vi "peg-in-hole Test with points and cloud.vi"() -> ()   [LabVIEW 2013]
uses:
  ROS/Code/SubVIs/BaxterSide.ctl
  <vilib>/Utility/config.llb/Read Key (String).vi
  Arm Globals.vi
  <vilib>/Utility/file.llb/Write To Spreadsheet File (DBL).vi
  <vilib>/Utility/config.llb/NI_LVConfig.lvlib
panel:
  out "time":dbl=251572.85700000002
  out "start":u32
  in  "Cloud File":path=path "C:/Program Files/Labview/user.lib/ROSforLV_0.1/Devices/Baxter/NIST2/Peg-in-hole/cloud.script"
  out "Array":cluster{dbl, dbl, dbl, dbl, dbl, dbl}[](array[cluster]) {"?" format="%.6f"}
  in  "Peg Size":dbl=3.0
  in  "Midpoint Name":string="hm"
  in  "h2 Name":string="h2"
  in  "h1 Name":string="h1"
  out "Times":dbl[](array[numeric]) format="%.1f"
  out "Status":string
  in  "Stop":bool
  out "error out":errorcluster
  # "as in Positions.cfg"
  # "Data is saved automatically at end of run\nSet peg size first"
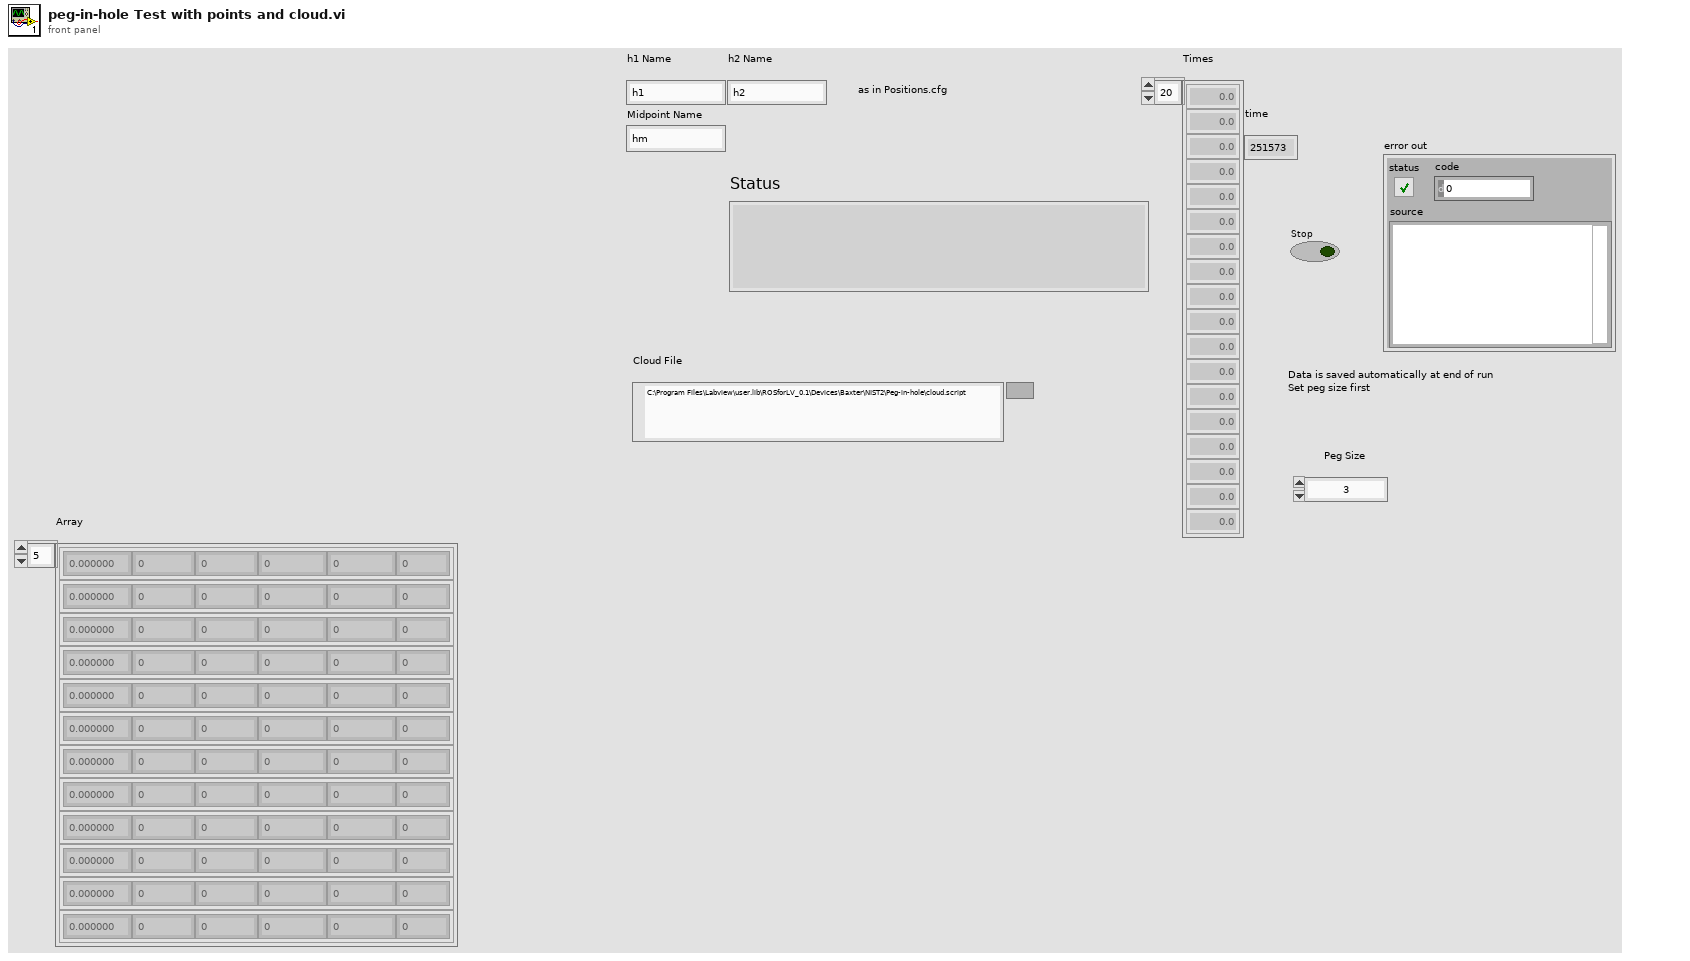
[diagram p1: front panel]
types:
  T1 = typedef "BaxterSide.ctl" = enum16{"left", "right"}
  T2 = typedef "NI_LVConfig.lvlib/Config Data RefNum.ctl" = refnum<k1>
  T3 = typedef "NI_Matrix.lvlib/RealMatrix.ctl" = dbl[][]
  T4 = cluster{"X":dbl, "Y":dbl, "Z":dbl, "Roll":dbl, "Pitch":dbl, "Yaw":dbl}
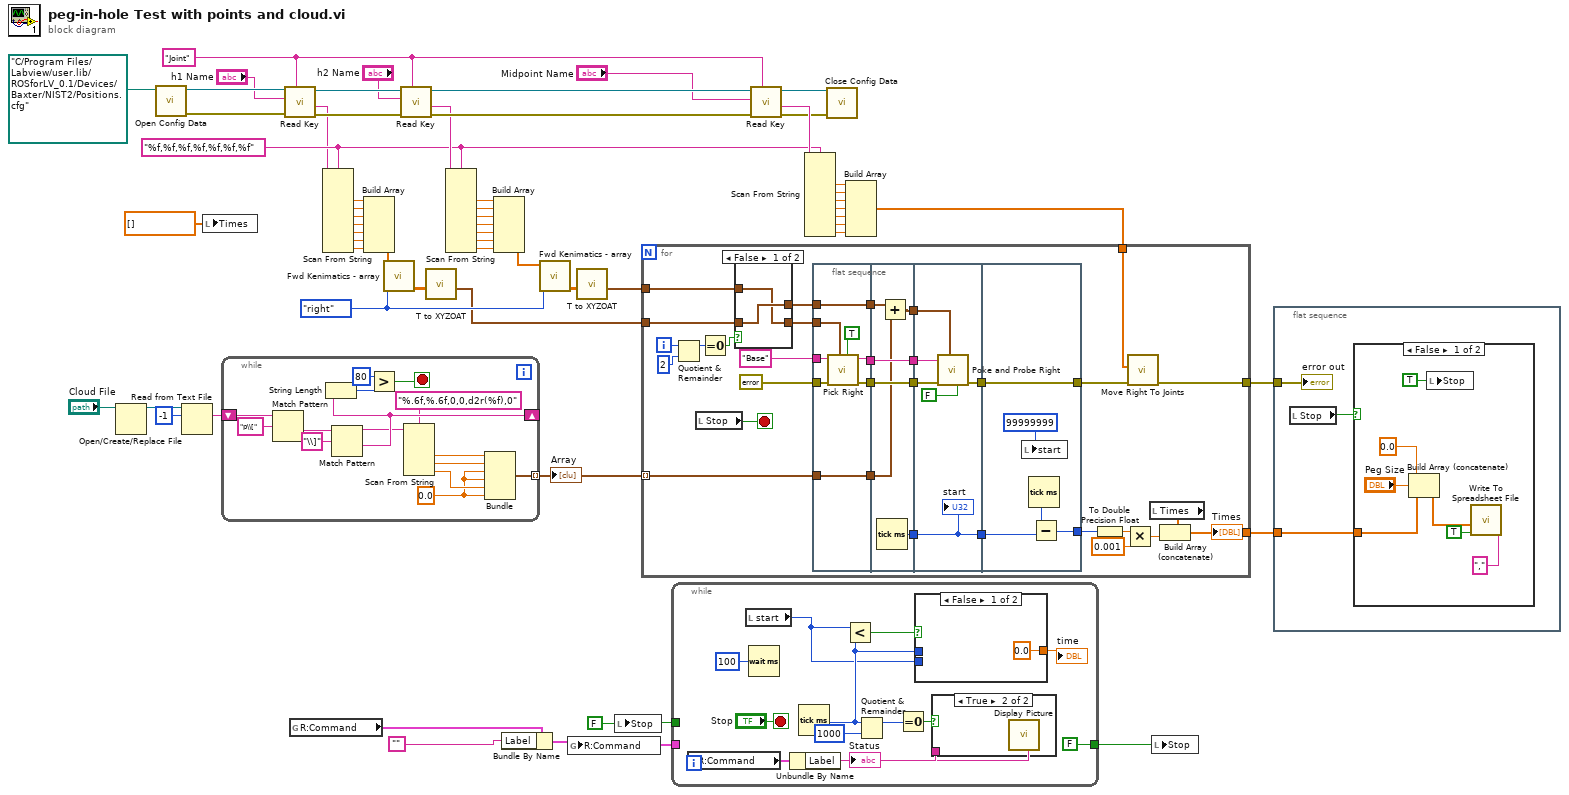
[diagram p0: block diagram]
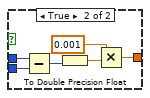
[diagram p3: hidden frame]
diagram:
  w31 = BaxterSide."right" ("Side")
  w15 = "%f,%f,%f,%f,%f,%f,%f" ("format string")
  w22 = "Joint" ("section")
  w58 = FALSE ("Stop")
  n1 = Open/Create/Replace File(file path (use dialog)="Cloud File") -> (refnum out=w5:refnum<file>)  [unwired: 5 in, 2 out]
  n2 = call <vilib>:"Open Config Data.vi"("configuration file path"=path "C:/Program Files/Labview/user.lib/ROSforLV_0.1/Devices/Baxter/NIST2/Positions.cfg") -> ("error out"=w51:errorcluster, "refnum"=w52:T2)  [unwired: 8 in, 1 out]
  n3 = Read from Text File(file (use dialog)=w5, count=-1) -> (text=w3:string)  [unwired: 2 in, 3 out]
  n4 = local write "Times"(dbl[] [] ("Times")) -> ()
  n5 = while {
    shift-right: [w68] -> _
    shift-left: w3 -> [w60]
    tunnel: [w64] -> w1 mode=indexing
    stop <- w72 stop-if-true
    w61 = 0.0
    n6 = Match Pattern(string=w60, regular expression="p\\[") -> (after substring=w70:string)  [unwired: 1 in, 3 out]
    n7 = Match Pattern(string=w70, regular expression="\\]") -> (before substring=w67:string, after substring=w68:string)  [unwired: 1 in, 2 out]
    n8 = String Length(string=w68) -> (length=w74:i32)
    n9 = Greater?(x=80, y=w74) -> (0:w72:bool)
    n10 = Scan From String(format string="%.6f,%.6f,0,0,d2r(%f),0", input string=w67) -> (output 1=w65:dbl, output 2=w63:dbl, output 3=w62:dbl)  [unwired: 5 in, 3 out]
    n11 = Bundle(w65, w63, w61, w61, w62, w61) -> (w64:cluster{dbl, dbl, dbl, dbl, dbl, dbl})  [unwired: 1 in]
  }
  "Array" <- w1
  n12 = call-poly <vilib>:"Read Key.vi"("section"=w22, "error in (no error)"=w51, "key"="h1 Name", "refnum"=w52) -> ("error out"=w25:errorcluster, "value"=w9:string, "refnum out"=w26:T2)  [unwired: 4 in, 1 out]
  n13 = global read "Arm Globals.vi" "R:Command"() -> (w54:cluster{"Label":string, "Angles":dbl[]})
  n14 = Scan From String(format string=w15, input string=w9) -> (output 1=w50:dbl, output 2=w49:dbl, output 3=w48:dbl, output 4=w47:dbl, output 5=w46:dbl, output 6=w45:dbl, output 7=w44:dbl)  [unwired: 9 in, 3 out]
  n15 = Build Array(w50, w49, w48, w47, w46, w45, w44) -> (w32:dbl[])
  n16 = call "Fwd Kenimatics - array.vi"("Side"=w31, "Joints"=w32) -> ("Matrix"=w30:T3)  [unwired: 8 in, 1 out]
  n17 = call-poly <vilib>:"Read Key.vi"("section"=w22, "error in (no error)"=w25, "key"="h2 Name", "refnum"=w26) -> ("error out"=w23:errorcluster, "value"=w16:string, "refnum out"=w24:T2)  [unwired: 4 in, 1 out]
  n18 = call "T to XYZOAT.vi"("T"=w30) -> ("XYZOAT"=w28:T4)  [unwired: 10 in]
  n19 = Scan From String(format string=w15, input string=w16) -> (output 1=w21:dbl, output 2=w20:dbl, output 3=w19:dbl, output 4=w18:dbl, output 5=w17:dbl, output 6=w12:dbl, output 7=w11:dbl)  [unwired: 9 in, 3 out]
  n20 = Build Array(w21, w20, w19, w18, w17, w12, w11) -> (w13:dbl[])
  n21 = Bundle By Name(cluster=w54, "Label"="") -> (w56:cluster{"Label":string, "Angles":dbl[]})
  n22 = call "Fwd Kenimatics - array.vi"("Side"=w31, "Joints"=w13) -> ("Matrix"=w29:T3)  [unwired: 8 in, 1 out]
  n23 = global write "Arm Globals.vi" "R:Command"(w56) -> ()
  n24 = call "T to XYZOAT.vi"("T"=w29) -> ("XYZOAT"=w27:T4)  [unwired: 10 in]
  n25 = local write "Stop"(w58) -> ()
  n26 = while {
    tunnel: w56 -> [_]
    tunnel: [FALSE] -> w57
    tunnel: w58 -> [_]
    stop <- "Stop" stop-if-true
    n27 = global read "Arm Globals.vi" "R:Command"() -> (w86:cluster{"Label":string, "Angles":dbl[]})
    n28 = local read "start"() -> (w77:u32)
    n29 = Wait (ms)(milliseconds to wait=u32 100) -> ()  [unwired: 1 out]
    n30 = Unbundle By Name(w86) -> ("Label"=w80:string)
    "Status" <- w80
    n31 = Tick Count (ms)() -> (millisecond timer value=w78:u32)
    n32 = Less?(x=w77, y=w78) -> (x < y?=w79:bool)
    n33 = Quotient & Remainder(x=w78, y=u32 1000) -> (x-y*floor(x/y)=w82:u32)  [unwired: 1 out]
    n34 = Equal To 0?(x=w82) -> (x = 0?=w81:bool)
    n35 = case shown="False" w79 {
      tunnel: w78 -> [_ w93]
      tunnel: w77 -> [_ w92]
      tunnel: [0.0 w88] -> w76
      frame False {
      }
      frame True {
        n36 = Subtract(x=w93, y=w92) -> (x-y=w91:u32)
        n37 = To Double Precision Float(number=w91) -> (double precision float=w90:dbl)
        n38 = Multiply(x=0.001, y=w90) -> (x*y=w88:dbl)
      }
    }
    "time" <- w76
    n39 = case shown="True" w81 {
      tunnel: w80 -> [_ w94]
      frame False {
      }
      frame True {
        n40 = call "Display Picture.vi"("Comment"=w94) -> ()  [unwired: 10 in, 1 out]
      }
    }
  }
  n41 = call-poly <vilib>:"Read Key.vi"("section"=w22, "error in (no error)"=w23, "key"="Midpoint Name", "refnum"=w24) -> ("error out"=w34:errorcluster, "value"=w36:string, "refnum out"=w35:T2)  [unwired: 4 in, 1 out]
  n42 = Scan From String(format string=w15, input string=w36) -> (output 1=w43:dbl, output 2=w42:dbl, output 3=w41:dbl, output 4=w40:dbl, output 5=w39:dbl, output 6=w38:dbl, output 7=w37:dbl)  [unwired: 9 in, 3 out]
  n43 = call <vilib>:"Close Config Data.vi"("error in (no error)"=w34, "refnum"=w35) -> ()  [unwired: 8 in, 2 out]
  n44 = Build Array(w43, w42, w41, w40, w39, w38, w37) -> (w14:dbl[])
  n45 = for {
    tunnel: [w106] -> w59
    tunnel: w27 -> [w118]
    tunnel: w28 -> [w119]
    tunnel: w14 -> [w100]
    tunnel: [w98] -> w6
    tunnel: w1 -> [w96] mode=indexing
    i -> [w123]
    stop <- w99 stop-if-true
    n46 = Quotient & Remainder(x=w123, y=2) -> (x-y*floor(x/y)=w121:i32)  [unwired: 1 out]
    n47 = local read "Stop"() -> (w99:bool)
    n48 = Equal To 0?(x=w121) -> (x = 0?=w120:bool)
    n49 = case shown="False" w120 {
      tunnel: w119 -> [w127 w129]
      tunnel: [w126 w129] -> w113
      tunnel: w118 -> [w126 w128]
      tunnel: [w127 w128] -> w111
      frame False {
      }
      frame True {
      }
    }
    n50 = flat-sequence {
      tunnel: "Base" ("Location Out") -> [w135]
      tunnel: errorcluster {"status"=FALSE, "code"=0, "source"=""} ("error in") -> [w137]
      tunnel: [w136] -> w117
      tunnel: [w134] -> w115
      tunnel: w113 -> [w133]
      tunnel: [w132] -> w112
      tunnel: w111 -> [w132]
      tunnel: [w131] -> w97
      tunnel: w96 -> [w131]
      tunnel: w117 -> [w143]
      tunnel: [w143] -> w116
      tunnel: w115 -> [w142]
      tunnel: [w142] -> w114
      tunnel: w112 -> [w140]
      tunnel: [w141] -> w108
      tunnel: w97 -> [w139]
      tunnel: [w138] -> w95
      tunnel: [w146] -> w110
      tunnel: w116 -> [w149]
      tunnel: w114 -> [w148]
      tunnel: [w145] -> w109
      tunnel: w108 -> [w145]
      tunnel: w95 -> [w147]
      tunnel: w110 -> [w152]
      tunnel: w109 -> [w153]
      tunnel: [w152] -> w107
      tunnel: [w151] -> w105
      frame #0 {
        n51 = call "Pick Right.vi"("Pause on Miss?"=TRUE, "Pick"=w133, "error in"=w137, "Location"=w135) -> ("error out"=w136:errorcluster, "Location Out"=w134:string)  [unwired: 6 in]
      }
      frame #1 {
        n52 = Tick Count (ms)() -> (millisecond timer value=w141:u32)
        n53 = Add(x=w140, y=w139) -> (x+y=w138:cluster{dbl, dbl, dbl, dbl, dbl, dbl})
      }
      frame #2 {
        n54 = call "Poke and Probe Right.vi"("Tap In?"=FALSE, "Goal"=w147, "error in"=w149, "Location"=w148) -> ("error out"=w146:errorcluster)  [unwired: 5 in, 2 out]
        "start" <- w145
      }
      frame #3 {
        n55 = local write "start"(u32 99999999 ("start")) -> ()
        n56 = Tick Count (ms)() -> (millisecond timer value=w154:u32)
        n57 = Subtract(x=w154, y=w153) -> (x-y=w151:u32)
      }
    }
    n58 = To Double Precision Float(number=w105) -> (double precision float=w104:dbl)
    n59 = Multiply(x=w104, y=0.001) -> (x*y=w101:dbl)
    n60 = call "Move Right To Joints.vi"("error in"=w107, "Goal"=w100) -> ("error out"=w106:errorcluster)  [unwired: 8 in, 1 out]
    n61 = local read "Times"() -> (w102:dbl[])
    n62 = Build Array (concatenate)(w102, w101) -> (w98:dbl[])
    "Times" <- w98
  }
  n63 = local write "Stop"(w57) -> ()
  n64 = flat-sequence {
    tunnel: w59 -> [w157]
    tunnel: w6 -> [w155]
    frame #0 {
      n65 = local read "Stop"() -> (w156:bool)
      n66 = case shown="False" w156 {
        tunnel: w155 -> [w161 _]
        frame False {
          n67 = Build Array (concatenate)(0.0 ("element"), "Peg Size", w161) -> (w159:dbl[])
          n68 = local write "Stop"(TRUE ("Stop")) -> ()
          n69 = call-poly <vilib>:"Write To Spreadsheet File.vi"("delimiter (\\t)"="," ("delimiter (\\t)"), "append to file? (new file:F)"=TRUE, "1D data"=w159) -> ()  [unwired: 5 in, 1 out]
        }
        frame True {
        }
      }
      "error out" <- w157
    }
  }
